vi "power conversion.vi"(8 "error in (no error)":errorcluster, 11 "AOTF in":refnum<class "AOTF.lvclass">) -> (0 "error out":errorcluster, 3 "AOTF out":refnum<class "AOTF.lvclass">)   [LabVIEW 2012, in "AOTF.lvclass"]
uses:
  AOTF.lvclass
  AOTF.lvclass/AOTF.ctl
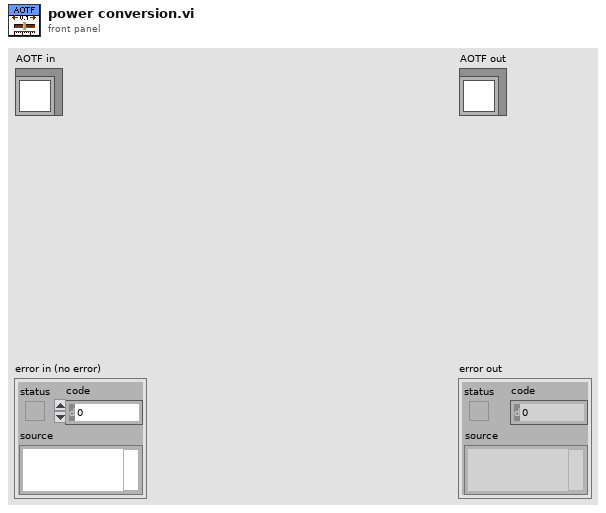
[diagram p1: front panel]
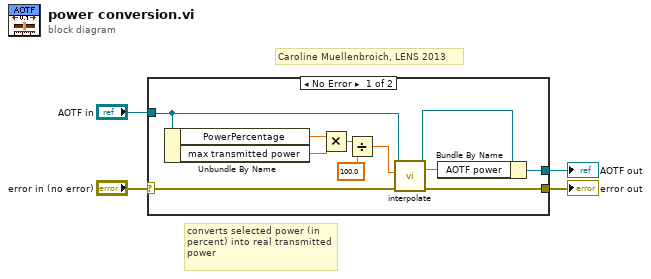
[diagram p0: block diagram]
diagram:
  # "converts selected power (in percent) into real transmitted power"
  # "Caroline Muellenbroich, LENS 2013"
  n1 = case shown="No Error" "error in (no error)" {
    selector: "error in (no error)" -> [w15 w17]
    tunnel: [w14 w17] -> w3
    tunnel: [w6 w16] -> w1
    tunnel: "AOTF in" -> [w5 w16]
    frame No Error {
      n2 = Unbundle By Name(w5) -> ("PowerPercentage"=w13:dbl, "max transmitted power"=w12:dbl)
      n3 = Multiply(x=w13, y=w12) -> (x*y=w11:dbl)
      n4 = Divide(x=w11, y=100.0) -> (x/y=w9:dbl)
      n5 = call-dynamic "interpolate.vi"("error in (no error)"=w15, "element in"=w9, "AOTF in"=w5) -> ("error out"=w14:errorcluster, "element out"=w8:dbl, "AOTF out"=w7:refnum<class "AOTF.lvclass">)  [unwired: 6 in]
      n6 = Bundle By Name(cluster=w7, "AOTF power"=w8) -> (w6:refnum<class "AOTF.lvclass">)
    }
    frame Error {
    }
  }
  "error out" <- w3
  "AOTF out" <- w1
